vi "Set Received Notifier.vi"(8 "error in":errorcluster, 10 "Received Notifier":refnum<notifier>, 11 "SDO Transfer in":refnum<class "SDO Transfer.lvclass">) -> (0 "error out":errorcluster, 3 "SDO Transfer out":refnum<class "SDO Transfer.lvclass">)   [LabVIEW 2020, in "SDO Manager.lvlib" / "SDO Transfer.lvclass"]
uses:
  SDO Transfer.lvclass
  SDO Transfer.lvclass/SDO Transfer.ctl
  Typedefs/SDO Result.ctl
  CANopen.lvlib
  SDO abort code.ctl
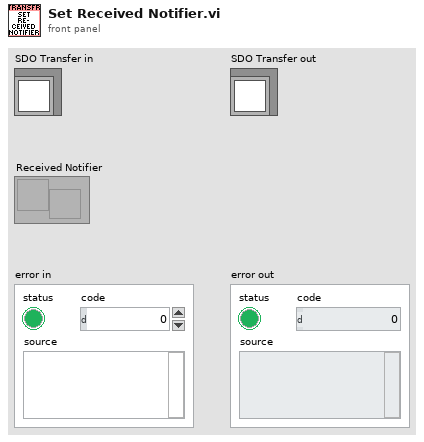
[diagram p1: front panel]
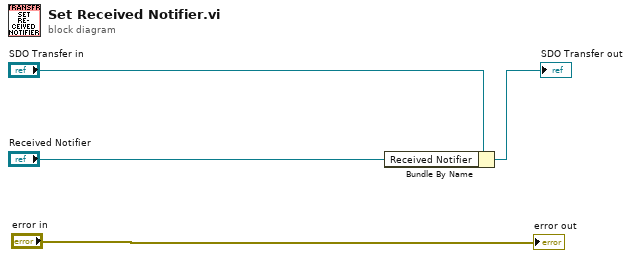
[diagram p0: block diagram]
diagram:
  n1 = Bundle By Name(cluster="SDO Transfer in", "Received Notifier"="Received Notifier") -> (→"SDO Transfer out":refnum<class "SDO Transfer.lvclass">)
  "error out" <- "error in"
